vi "Part 1.vi"(11 "Input":string) -> (3 "Output":i64)   [LabVIEW 2021]
uses:
  <userlib>/_OpenG.lib/string/string.llb/Convert EOLs (String)__ogtk.vi
panel:
  out "array 2":string[](array[string])
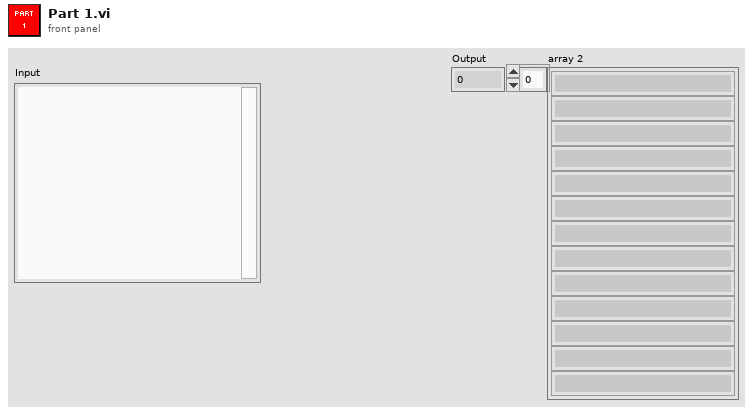
[diagram p1: front panel]
types:
  T1 = map{string, cluster{"Left":string, "Right":string}}
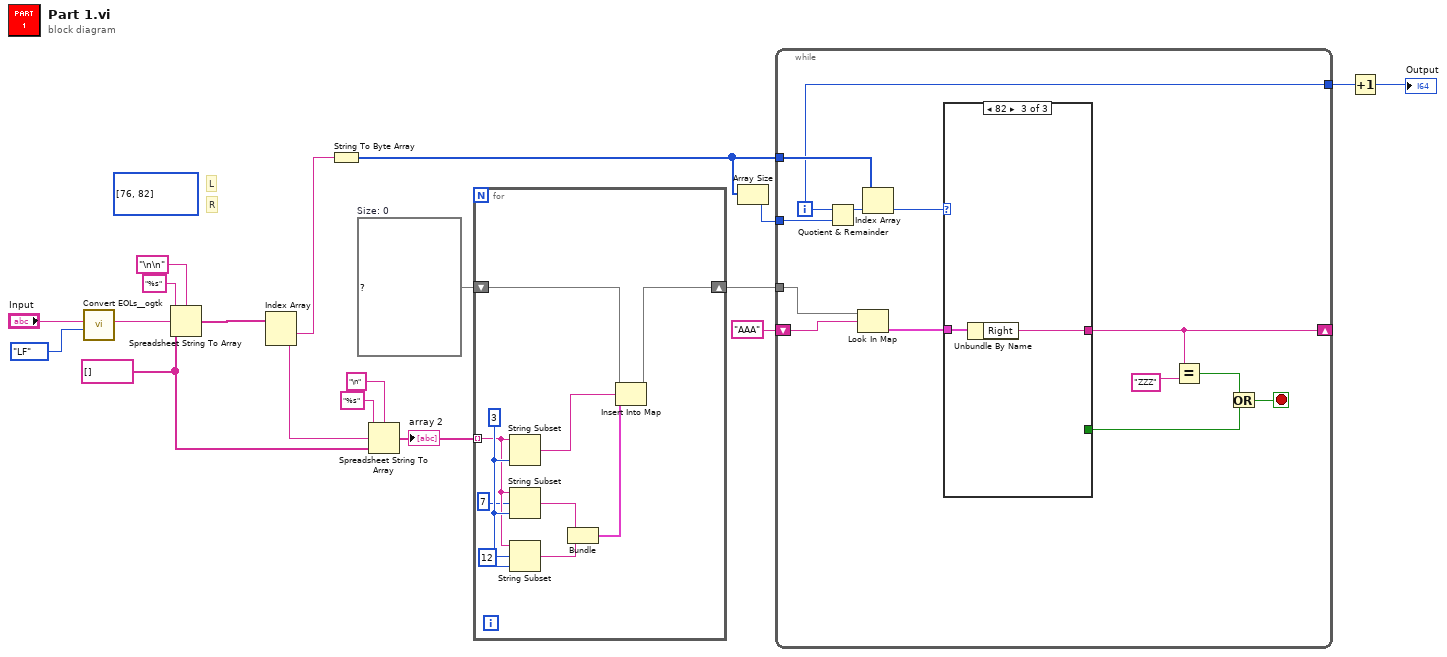
[diagram p0: block diagram]
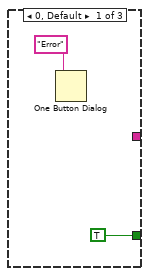
[diagram p2: hidden frame]
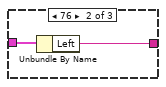
[diagram p3: hidden frame]
diagram:
  w7 = T1 {}  # Size: 0
  (unwired) u8[] [76, 82] ("unsigned byte array")
  w9 = string[] []
  # "R"
  # "L"
  n1 = call-poly <userlib>:"Convert EOLs__ogtk.vi"("Convert to:"=enum16{"CR", "LF", "CRLF"}."LF", "String in"="Input") -> ("String out"=w16:string)  [unwired: 9 in]
  n2 = Spreadsheet String To Array(delimiter (Tab)="\n\n", format string="%s", spreadsheet string=w16, array type (2D Dbl)=w9) -> (array=w14:string[])
  n3 = Index Array(array=w14) -> (element #1=w13:string, element #2=w10:string)  [unwired: 2 in]
  n4 = String To Byte Array(string=w13) -> (unsigned byte array=w5:u8[])
  n5 = Spreadsheet String To Array(delimiter (Tab)="\n", format string="%s", spreadsheet string=w10, array type (2D Dbl)=w9) -> (array=w8:string[])
  "array 2" <- w8
  n6 = for {
    tunnel: w8 -> [w28] mode=indexing
    shift-right: [w20] -> w6
    shift-left: w7 -> [w22]
    w29 = 3
    n7 = String Subset(string=w28, length (rest)=w29) -> (substring=w23:string)  [unwired: 1 in]
    n8 = String Subset(string=w28, offset (0)=7, length (rest)=w29) -> (substring=w24:string)
    n9 = String Subset(string=w28, offset (0)=12, length (rest)=w29) -> (substring=w25:string)
    n10 = Bundle(w24, w25) -> (w21:cluster{string, string})  [unwired: 1 in]
    n11 = Insert Into Map(map in=w22, key=w23, value=w21) -> (map out=w20:T1)  [unwired: 2 out]
  }
  n12 = Array Size(array=w5) -> (size(s)=w4:i32)
  n13 = while {
    tunnel: w4 -> [w42]
    tunnel: w5 -> [w40]
    shift-right: [w35] -> _
    shift-left: "AAA" -> [w37]
    tunnel: w6 -> [w38]
    tunnel: [w30] -> w2
    i -> [w30]
    stop <- w31 stop-if-true
    n14 = Quotient & Remainder(x=w30, y=w42) -> (x-y*floor(x/y)=w41:i32)  [unwired: 1 out]
    n15 = Look In Map(map=w38, key=w37) -> (value=w36:cluster{"Left":string, "Right":string})  [unwired: 1 in, 1 out]
    n16 = Index Array(array=w40, index=w41) -> (element=w39:u8)
    n17 = case shown="82" w39 {
      tunnel: w36 -> [_ w46 w48]
      tunnel: [_ w45 w47] -> w35
      tunnel: [TRUE _ _] -> w32
      frame 0, Default {
        n18 = One Button Dialog(message="Error") -> ()  [unwired: 1 in, 1 out]
      }
      frame 76 {
        n19 = Unbundle By Name(w46) -> ("Left"=w45:string)
      }
      frame 82 {
        n20 = Unbundle By Name(w48) -> ("Right"=w47:string)
      }
    }
    n21 = Equal?(x=w35, y="ZZZ") -> (x = y?=w33:bool)
    n22 = Or(x=w33, y=w32) -> (x .or. y?=w31:bool)
  }
  n23 = Increment(x=w2) -> (x+1=→"Output":i32)
